vi "mod_Passband PLL.vi"(0 "passband waveform":waveform(dbl)={"t0"=timestamp(0 s since 1904-01-01), "dt"=0.0, "Y"=[]}, 1 "loop filter (reverse coefficients)":dbl[](array[numeric])=[1.0, -1.0], 5 "VCO carrier frequency (Hz)":dbl, 7 "VCO initial phase (degrees)":dbl, 9 "VCO gain (degrees/V)":dbl=1.0 format="%#_6p", 11 "error in (no error)":errorcluster, 12 "loop filter (forward coefficients)":dbl[](array[numeric])=[1.05, -0.95], 13 "reset ?(T)":bool=TRUE) -> (4 "VCO phase (degrees)":dbl[](array[numeric]), 6 "phase error (degrees)":dbl[](array[numeric]), 8 "estimated carrier frequency (Hz)":dbl, 10 "estimated initial phase (degrees)":dbl, 15 "error out":errorcluster)   [LabVIEW 2020, in "niAMT.lvlib"]
uses:
  <vilib>/addons/Modulation/niAMT.lvlib
  <vilib>/addons/Modulation/Analog/controls/Complex Data Waveform.ctl
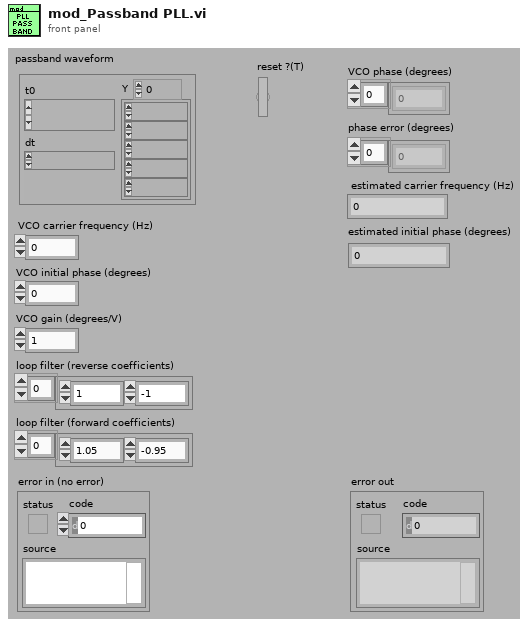
[diagram p1: front panel]
types:
  T1 = typedef "niAMT.lvlib/Complex Data Waveform.ctl" = cluster{"t0":dbl, "dt":dbl, "Y":cdb[]}
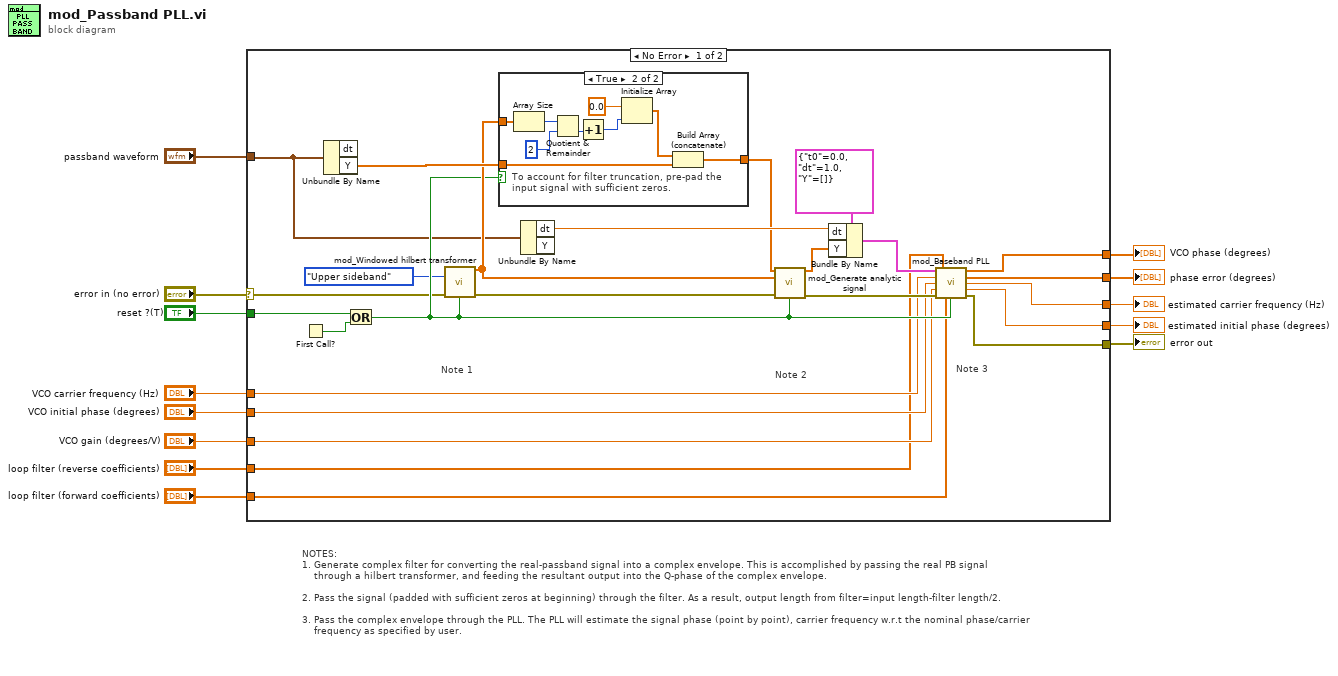
[diagram p0: block diagram]
diagram:
  # "NOTES:\n1. Generate complex filter for converting the real-passband signal into a complex envelope. This is accomplished by passing the real PB signal\n    through a hilbert transformer, and feeding the resultant output into the Q-phase of the complex envelope.\n\n2. Pass the signal (padded with sufficient zeros at beginning) through the filter. As a result, output length from filter=input length-filter length/2.\n\n3. Pass the complex envelope through the PLL. The PLL will estimate the signal phase (point by point), carrier frequency w.r.t the nominal phase/carrier\n    frequency as specified by user."
  n1 = case shown="No Error" "error in (no error)" {
    selector: "error in (no error)" -> [w27 w49]
    tunnel: "reset ?(T)" -> [w38 _]
    tunnel: "passband waveform" -> [w28 _]
    tunnel: [w26 w49] -> w10
    tunnel: "VCO carrier frequency (Hz)" -> [w25 _]
    tunnel: "VCO initial phase (degrees)" -> [w24 _]
    tunnel: "VCO gain (degrees/V)" -> [w23 _]
    tunnel: "loop filter (reverse coefficients)" -> [w22 _]
    tunnel: "loop filter (forward coefficients)" -> [w21 _]
    tunnel: [w20 _] -> w4
    tunnel: [w19 _] -> w3
    tunnel: [w18 _] -> w2
    tunnel: [w17 _] -> w1
    frame No Error {
      # "Note 3"
      # "Note 2"
      # "Note 1"
      n2 = First Call?() -> (First Call?: T/F=w37:bool)
      n3 = Unbundle By Name(w28) -> ("Y"=w36:dbl[])  [unwired: 1 out]
      n4 = Or(x=w38, y=w37) -> (x .or. y?=w29:bool)
      n5 = call <vilib>:"mod_Windowed hilbert transformer.vi"("side-band"=enum16{"Lower sideband", "Upper sideband"}."Upper sideband", "error in (no error)"=w27, "reset? (T)"=w29) -> ("hilbert transformer taps"=w34:cdb[], "error out"=w35:errorcluster)  [unwired: 1 in, 10 out]
      n6 = case shown="True" w29 {
        tunnel: w36 -> [w39 w48]
        tunnel: w34 -> [_ w47]
        tunnel: [w39 w42] -> w16
        frame False {
        }
        frame True {
          # "To account for filter truncation, pre-pad the\ninput signal with sufficient zeros."
          n7 = Array Size(array=w47) -> (size(s)=w41:i32)
          n8 = Quotient & Remainder(x=w41, y=2) -> (floor(x/y)=w45:i32)  [unwired: 1 out]
          n9 = Increment(x=w45) -> (x+1=w40:i32)
          n10 = Initialize Array(0.0 ("element"), w40) -> (w43:dbl[])
          n11 = Build Array (concatenate)(w43, w48) -> (w42:dbl[])
        }
      }
      n12 = Unbundle By Name(w28) -> ("dt"=w31:dbl)  [unwired: 1 out]
      n13 = call <vilib>:"mod_Generate analytic signal.vi"("m(t)"=w16, "filter taps"=w34, "error in (no error)"=w35, "reset? (T)"=w29) -> ("analytic signal"=w14:cdb[], "error out"=w33:errorcluster)  [unwired: 10 out]
      n14 = Bundle By Name(cluster=T1 {"t0"=0.0, "dt"=1.0, "Y"=[]} ("input complex waveform"), "dt"=w31, "Y"=w14) -> (w30:T1)
      n15 = call <vilib>:"mod_Baseband PLL.vi"("baseband waveform (complex)"=w30, "loop filter (reverse coefficients)"=w22, "VCO carrier frequency (Hz)"=w25, "VCO initial phase (degrees)"=w24, "VCO gain (degrees/V)"=w23, "error in (no error)"=w33, "loop filter (forward coefficients)"=w21, "reset ?(T)"=w29) -> ("VCO phase (degrees)"=w20:dbl[], "phase error (degrees)"=w17:dbl[], "estimated carrier frequency (Hz)"=w19:dbl, "estimated initial phase (degrees)"=w18:dbl, "error out"=w26:errorcluster)  [unwired: 3 out]
    }
    frame Error {
    }
  }
  "error out" <- w10
  "estimated initial phase (degrees)" <- w2
  "phase error (degrees)" <- w1
  "estimated carrier frequency (Hz)" <- w3
  "VCO phase (degrees)" <- w4
